vi "Disconnect SMU Resources from site - 4163 only.vi"(0 "TSM context":T1, 11 "error in":errorcluster) -> (4 "TSM context out":T1, 15 "error out":errorcluster)   [LabVIEW 2019]
doc: "This VI is used to disconnect SMU resources safely by preventing potetial OCP errors."
uses:
  <vilib>/NI_TestStand_SemiconductorModule/NI_TestStand_Semiconductor_Module.lvlibp/PinMap/General/SemiconductorModuleContext.ctl
  <instrlib>/niDCPower/nidcpower.llb/niDCPower Sense.ctl
  <instrlib>/niDCPower/nidcpower.llb/niDCPower Output Function.ctl
  <vilib>/Utility/High Resolution Polling Wait.vi
  SSC DCPower/Source/SSC DCPower Configure Output Connected.vi
  SSC DCPower/Source/SSC DCPower Configure Output Enabled.vi
  <vilib>/NI_TestStand_SemiconductorModule/NI_TestStand_Semiconductor_Module.lvlibp
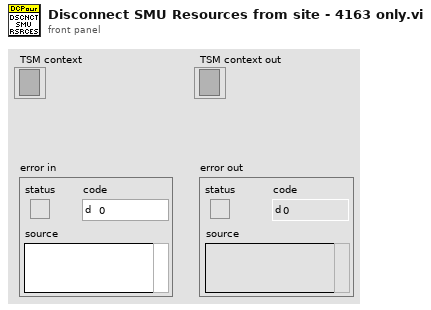
[diagram p1: front panel]
types:
  T1 = typedef "NI_TestStand_Semiconductor_Module.lvlibp/SemiconductorModuleContext.ctl" = refnum<k7>
  T2 = typedef "niDCPower Output Function.ctl" = i32
  T3 = typedef "niDCPower Sense.ctl" = i32
  T4 = typedef "TSM SSC DCPower.ctl" = cluster{"Pin Query Context":refnum<class "MultiplePinMultipleSessionQueryContext.lvclass">, "SSC":T5[], "Site Numbers":i32[], "Pins":T6[], "Pins Expanded":T8[]}
  T5 = typedef "SSC DCPower.ctl" = cluster{"Session":refnum<k15>, "Chan":string, "Channel List":string}
  T6 = typedef "TSM Pin Information.ctl" = cluster{"Pin":tag, "Type":T7, "Count":i32}
  T7 = typedef "TSM Pin Type Identifier.ctl" = enum8{"DUT Pin", "System Pin", "Pin Group", "Not Determined"}
  T8 = typedef "TSM Expanded Pin Information.ctl" = cluster{"Pin":tag, "Type":T7, "Index":i32}
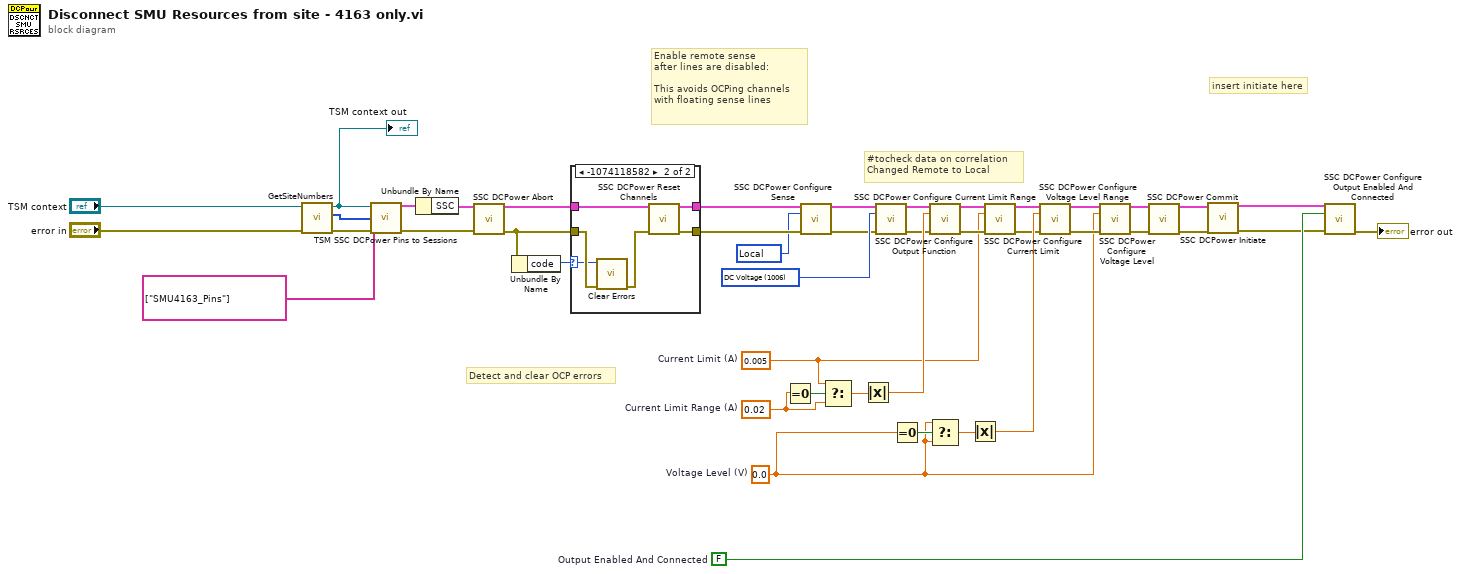
[diagram p0: block diagram]
diagram:
  w15 = T2 1006 items=["DC Voltage"=1006, "DC Current"=1007, "Pulse Voltage"=1049, "Pulse Current"=1050] ("Output Function")
  w14 = 0.005  # Current Limit (A)
  w12 = 0.0  # Voltage Level (V)
  w13 = 0.02  # Current Limit Range (A)
  w32 = T3 1008 items=["Local"=1008, "Remote"=1009] ("Sense")
  w37 = FALSE  # Output Enabled And Connected
  # "#tocheck data on correlation\nChanged Remote to Local"
  # "insert initiate here"
  # "Enable remote sense\nafter lines are disabled:\n\nThis avoids OCPing channels\nwith floating sense lines"
  # "Detect and clear OCP errors"
  n1 = call <vilib>:"GetSiteNumbers.vi"("error in (no error)"="error in", "Semiconductor Module Context"="TSM context") -> ("error out"=w35:errorcluster, "Site Numbers"=w33:i32[], "Semiconductor Module Context Out"=w34:T1)  [unwired: 6 in, 1 out]
  "TSM context out" <- w34
  n2 = call "TSM SSC DCPower Pins to Sessions.vi"("TSM context"=w34, "Pins"=tag[] ["SMU4163_Pins"], "Site Numbers"=w33, "error in"=w35) -> ("DCPower TSM Out"=w40:T4, "error out"=w9:errorcluster)  [unwired: 10 in]
  n3 = Unbundle By Name(w40) -> ("SSC"=w8:T5[])
  n4 = call "SSC DCPower Abort.vi"("DCPower SSC in"=w8, "error in"=w9) -> ("DCPower SSC out"=w39:T5[], "error out"=w42:errorcluster)  [unwired: 12 in]
  n5 = Unbundle By Name(w42) -> ("code"=w43:i32)
  n6 = case shown="-1074118582" w43 {
    selector: w43 -> [_ w48]
    tunnel: [w45 w50] -> w41
    tunnel: w42 -> [w45 w51]
    tunnel: w39 -> [w44 w47]
    tunnel: [w44 w46] -> w38
    frame Default {
    }
    frame -1074118582 {
      n7 = call <vilib>:"Clear Errors.vi"("error in (no error)"=w51, "specific error code to clear (0: all)"=w48) -> ("error out"=w49:errorcluster)  [unwired: 4 in, 1 out]
      n8 = call "SSC DCPower Reset Channels.vi"("DCPower SSC in"=w47, "error in"=w49) -> ("DCPower SSC out"=w46:T5[], "error out"=w50:errorcluster)  [unwired: 12 in]
    }
  }
  n9 = Equal To 0?(x=w13) -> (x = 0?=w30:bool)
  n10 = call "SSC DCPower Configure Sense.vi"("DCPower SSC in"=w38, "Sense"=w32, "error in"=w41) -> ("DCPower SSC out"=w10:T5[], "error out"=w11:errorcluster)  [unwired: 11 in]
  n11 = Select(t=w14, s=w30, f=w13) -> (s? t:f=w29:dbl)
  n12 = Absolute Value(x=w29) -> (abs(x)=w31:dbl)
  n13 = call "SSC DCPower Configure Output Function.vi"("DCPower SSC in"=w10, "Output Function"=w15, "error in"=w11) -> ("DCPower SSC out"=w16:T5[], "error out"=w17:errorcluster)  [unwired: 11 in]
  n14 = Equal To 0?(x=w12) -> (x = 0?=w26:bool)
  n15 = call "SSC DCPower Configure Current Limit Range.vi"("DCPower SSC in"=w16, "Current Limit Range (A)"=w31, "error in"=w17) -> ("DCPower SSC out"=w18:T5[], "error out"=w19:errorcluster)  [unwired: 11 in]
  n16 = Select(t=w12, s=w26, f=w12) -> (s? t:f=w27:dbl)
  n17 = Absolute Value(x=w27) -> (abs(x)=w28:dbl)
  n18 = call "SSC DCPower Configure Current Limit.vi"("DCPower SSC in"=w18, "Current Limit (A)"=w14, "error in"=w19) -> ("DCPower SSC out"=w20:T5[], "error out"=w21:errorcluster)  [unwired: 11 in]
  n19 = call "SSC DCPower Configure Voltage Level Range.vi"("DCPower SSC in"=w20, "Voltage Level Range (V)"=w28, "error in"=w21) -> ("DCPower SSC out"=w22:T5[], "error out"=w23:errorcluster)  [unwired: 11 in]
  n20 = call "SSC DCPower Configure Voltage Level.vi"("DCPower SSC in"=w22, "Voltage Level (V)"=w12, "error in"=w23) -> ("DCPower SSC out"=w25:T5[], "error out"=w24:errorcluster)  [unwired: 11 in]
  n21 = call "SSC DCPower Commit.vi"("DCPower SSC in"=w25, "error in"=w24) -> ("DCPower SSC out"=w7:T5[], "error out"=w5:errorcluster)  [unwired: 12 in]
  n22 = call "SSC DCPower Initiate.vi"("DCPower SSC in"=w7, "error in"=w5) -> ("DCPower SSC out"=w6:T5[], "error out"=w4:errorcluster)  [unwired: 12 in]
  n23 = call "SSC DCPower Configure Output Enabled And Connected.vi"("DCPower SSC in"=w6, "Output Enabled And Connected"=w37, "error in"=w4) -> ("error out"=→"error out":errorcluster)  [unwired: 11 in, 1 out]
